vi "Pcre2PatternInfo8.vi"(8 "error in":errorcluster, 10 "What":u32 format="%.0x", 11 "pCode":u64 format="%.0x") -> (0 "error out":errorcluster, 2 "Info":u32, 3 "pCode":u64 format="%.0x")   [LabVIEW 2021, in "libpcre2-8.lvlib"]
uses:
  libpcre2-8.lvlib
  libpcre2-8-x32.dll
panel:
  out "Pointer":u64
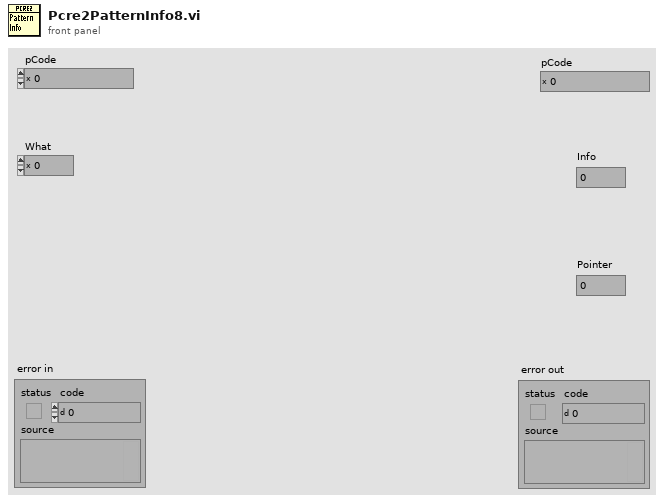
[diagram p1: front panel]
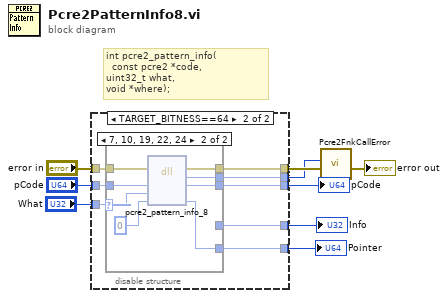
[diagram p0: block diagram]
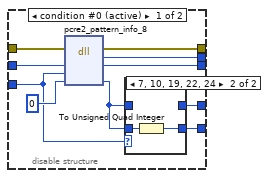
[diagram p2: hidden frame]
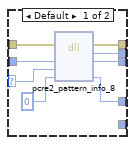
[diagram p4: hidden frame]
diagram:
  # "int pcre2_pattern_info(\n  const pcre2 *code,\nuint32_t what,\nvoid *where);"
  n1 = disable-structure shown="TARGET_BITNESS==64" {
    disable-tunnel: [w19 w30] -> w9
    disable-tunnel: [w10 w29] -> w8
    disable-tunnel: [w18 w28] -> w7
    disable-tunnel: [w17 w27] -> w5
    disable-tunnel: "error in" -> [w16 w26]
    disable-tunnel: "pCode" -> [w15 w25]
    disable-tunnel: "What" -> [w13 w24]
    disable-tunnel: [w12 w23] -> w1
    frame condition #0 (active) {
      n2 = dll-call lib="libpcre2-8-x*.dll" fn="pcre2_pattern_info_8"(error in=w16, "code"=w15, "what"=w13, "where"=u32 0) -> (error out=w18:errorcluster, "return type"=w17:i32, "code"=w19:u64, "where"=w11:u32)  [unwired: 3 in, 1 out]
      n3 = case shown="7, 10, 19, 22, 24" w13 {
        tunnel: w11 -> [_ w22]
        tunnel: [_ w21] -> w12
        tunnel: w11 -> [w20 _]
        tunnel: [w20 _] -> w10
        frame Default {
        }
        frame 7, 10, 19, 22, 24 {
          n4 = To Unsigned Quad Integer(1:w22) -> (0:w21:u64)
        }
      }
    }
    frame condition #1 {
      n5 = case shown="7, 10, 19, 22, 24" w24 {
        selector: w24 -> [w31 w40]
        tunnel: [w38 w46] -> w30
        tunnel: [w37 _] -> w29
        tunnel: [w36 w45] -> w28
        tunnel: [w35 w44] -> w27
        tunnel: w26 -> [w34 w43]
        tunnel: w25 -> [w32 w41]
        tunnel: [_ w39] -> w23
        frame Default {
          n6 = dll-call lib="libpcre2-8-x*.dll" fn="pcre2_pattern_info_8"(error in=w34, "code"=w32, "what"=w31, "where"=u32 0) -> (error out=w36:errorcluster, "return type"=w35:i32, "code"=w38:u64, "where"=w37:u32)  [unwired: 3 in, 1 out]
        }
        frame 7, 10, 19, 22, 24 {
          n7 = dll-call lib="libpcre2-8-x*.dll" fn="pcre2_pattern_info_8"(error in=w43, "code"=w41, "what"=w40, "where"=u64 0) -> (error out=w45:errorcluster, "return type"=w44:i32, "code"=w46:u64, "where"=w39:u64)  [unwired: 3 in, 1 out]
        }
      }
    }
  }
  "pCode" <- w9
  "Info" <- w8
  "Pointer" <- w1
  n8 = call "Pcre2FnkCallError.vi"("error in"=w7, "ErrorCode"=w5) -> ("error out"=→"error out":errorcluster)  [unwired: 9 in]
